vi "while_f_to_c.vi"() -> ()   [LabVIEW 2025]
panel:
  in  "Numeric 5":dbl
  in  "Numeric 4":dbl
  in  "Slide 2":dbl(slide) scale=0.0..200.0
  in  "stop 2":bool
  out "Numeric 3":i32
  out "Thermometer 2":dbl(slide) scale=0.0..200.0
  in  "Boolean":bool
  out "Thermometer":dbl(slide) scale=0.0..200.0
  out "Numeric 2":i32
  in  "stop":bool
  in  "Slide":dbl(slide) scale=0.0..200.0
  in  "Numeric":dbl
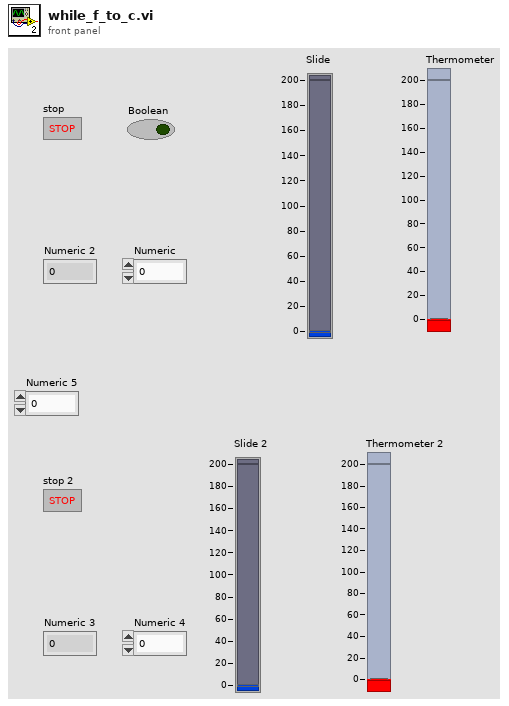
[diagram p1: front panel]
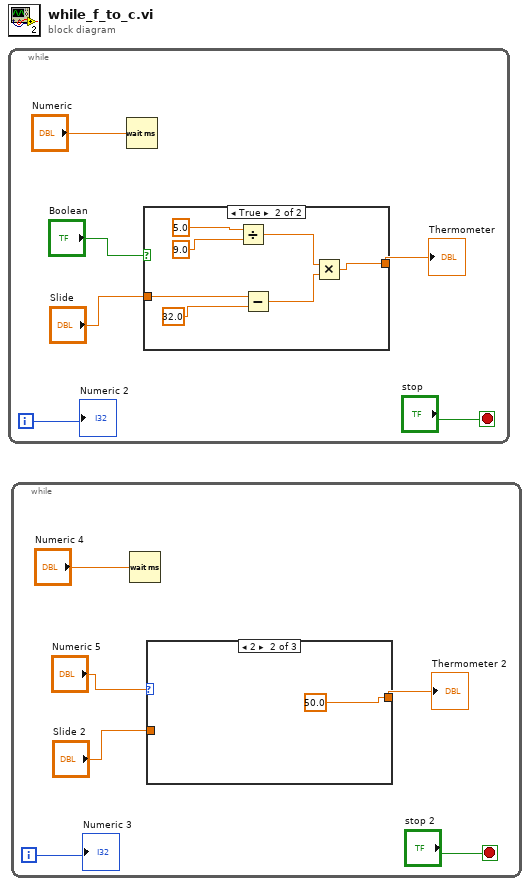
[diagram p0: block diagram]
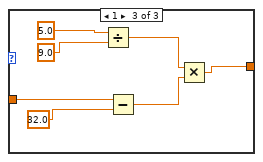
[diagram p3: hidden frame]
diagram:
  n1 = while {
    i -> [w5]
    stop <- "stop" stop-if-true
    n2 = Wait (ms)(milliseconds to wait="Numeric") -> ()  [unwired: 1 out]
    n3 = case shown="True" "Boolean" {
      tunnel: "Slide" -> [w7 w12]
      tunnel: [w7 w8] -> w2
      frame False {
      }
      frame True {
        n4 = Divide(x=5.0, y=9.0) -> (x/y=w10:dbl)
        n5 = Subtract(x=w12, y=32.0) -> (x-y=w9:dbl)
        n6 = Multiply(x=w10, y=w9) -> (x*y=w8:dbl)
      }
    }
    "Thermometer" <- w2
    "Numeric 2" <- w5
  }
  n7 = while {
    i -> [w19]
    stop <- "stop 2" stop-if-true
    n8 = Wait (ms)(milliseconds to wait="Numeric 4") -> ()  [unwired: 1 out]
    n9 = case shown="2" "Numeric 5" {
      tunnel: "Slide 2" -> [w21 _ w27]
      tunnel: [w21 50.0 ("Slide 2") w23] -> w16
      frame 0, Default {
      }
      frame 2 {
      }
      frame 1 {
        n10 = Divide(x=5.0, y=9.0) -> (x/y=w25:dbl)
        n11 = Subtract(x=w27, y=32.0) -> (x-y=w24:dbl)
        n12 = Multiply(x=w25, y=w24) -> (x*y=w23:dbl)
      }
    }
    "Thermometer 2" <- w16
    "Numeric 3" <- w19
  }
